vi "Saturation Move Sequence.vi"(2 "error in (no error)":errorcluster, 3 "Saturation Sweep Speed":dbl=2.0, 4 "Saturation End Angle":dbl=320.0, 5 ".NET Refnum in":refnum<k24>) -> (0 "error out":errorcluster, 1 "reference out":refnum<k24>)   [LabVIEW 2023]
uses:
  C:/Users/nanometa/Documents/TCSPC_Git_Repo/Source/ThorLabs.MotionControl.KCube.DCServoCLI.dll
  ThorLabs.MotionControl.KCube.DCServoCLI.dll
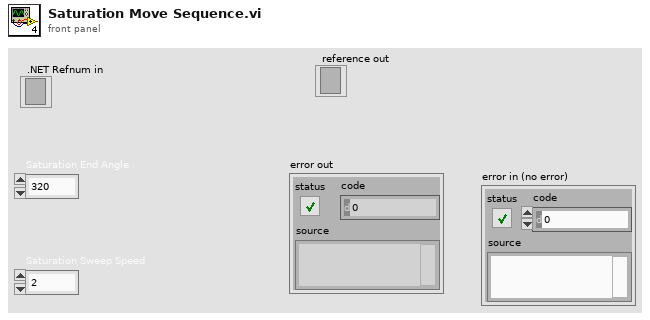
[diagram p1: front panel]
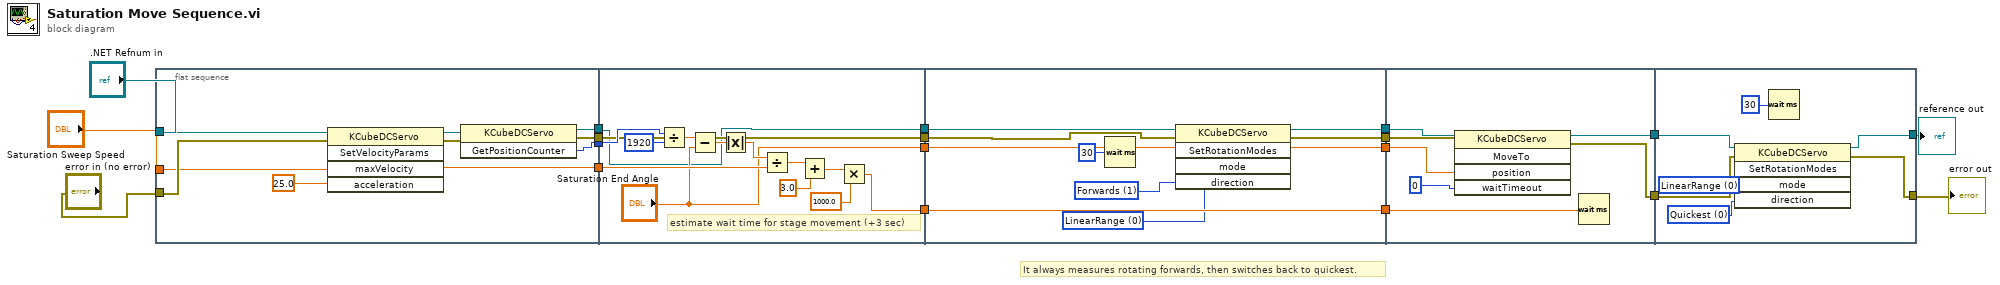
[diagram p0: block diagram]
diagram:
  # "It always measures rotating forwards, then switches back to quickest."
  n1 = flat-sequence {
    tunnel: [w27] -> w19
    tunnel: [w21] -> w18
    tunnel: [w25] -> w17
    tunnel: [w23] -> w16
    tunnel: "error in (no error)" -> [w22]
    tunnel: "Saturation Sweep Speed" -> [w21]
    tunnel: ".NET Refnum in" -> [w20]
    tunnel: w19 -> [w33]
    tunnel: w18 -> [w38]
    tunnel: [w32] -> w10
    tunnel: w17 -> [w32]
    tunnel: [w31] -> w8
    tunnel: ["Saturation End Angle"] -> w6
    tunnel: [w29] -> w4
    tunnel: w16 -> [w29]
    tunnel: w10 -> [w46]
    tunnel: [w47] -> w9
    tunnel: w8 -> [w51]
    tunnel: [w51] -> w7
    tunnel: w6 -> [w50]
    tunnel: [w50] -> w5
    tunnel: w4 -> [w49]
    tunnel: [w48] -> w3
    tunnel: w9 -> [w57]
    tunnel: w7 -> [w56]
    tunnel: w5 -> [w55]
    tunnel: w3 -> [w54]
    tunnel: [w53] -> w2
    tunnel: [w52] -> w1
    tunnel: [w60] -> w14
    tunnel: [w61] -> w15
    tunnel: w2 -> [w65]
    tunnel: w1 -> [w64]
    frame #0 {
      n2 = invoke class="KCubeDCServo" method="SetVelocityParams"(reference=w20, error in=w22, "maxVelocity"=w21, "acceleration"=25.0) -> (reference out=w24:refnum<k24>, error out=w26:errorcluster)  [unwired: 1 in, 3 out]
      n3 = invoke class="KCubeDCServo" method="GetPositionCounter"(reference=w24, error in=w26) -> (reference out=w23:refnum<k24>, error out=w25:errorcluster, "GetPositionCounter"=w27:i32)  [unwired: 1 in]
    }
    frame #1 {
      # "estimate wait time for stage movement (+3 sec)"
      n4 = Divide(x=w33, y=1920) -> (x/y=w41:dbl)
      n5 = Subtract(x=w41, y="Saturation End Angle") -> (x-y=w42:dbl)
      n6 = Absolute Value(x=w42) -> (abs(x)=w39:dbl)
      n7 = Divide(x=w39, y=w38) -> (x/y=w37:dbl)
      n8 = Add(x=w37, y=3.0) -> (x+y=w35:dbl)
      n9 = Multiply(x=w35, y=1000.0) -> (x*y=w31:dbl)
    }
    frame #2 {
      w43 = i16 0 items=["LinearRange", "RotationalUnlimited", "RotationalRange"] ("mode")
      w45 = i16 1 items=["Quickest", "Forwards", "Reverse"] ("direction")
      n10 = Wait (ms)(milliseconds to wait=u32 30) -> ()  [unwired: 1 out]
      n11 = invoke class="KCubeDCServo" method="SetRotationModes"(reference=w49, error in=w46, "mode"=w43, "direction"=w45) -> (reference out=w48:refnum<k24>, error out=w47:errorcluster)  [unwired: 1 in, 3 out]
    }
    frame #3 {
      n12 = invoke class="KCubeDCServo" method="MoveTo"(reference=w54, error in=w57, "position"=w55, "waitTimeout"=0) -> (reference out=w53:refnum<k24>, error out=w52:errorcluster)  [unwired: 1 in, 3 out]
      n13 = Wait (ms)(milliseconds to wait=w56) -> ()  [unwired: 1 out]
    }
    frame #4 {
      w59 = i16 0 items=["LinearRange", "RotationalUnlimited", "RotationalRange"] ("mode")
      w63 = i16 0 items=["Quickest", "Forwards", "Reverse"] ("direction")
      n14 = invoke class="KCubeDCServo" method="SetRotationModes"(reference=w65, error in=w64, "mode"=w59, "direction"=w63) -> (reference out=w61:refnum<k24>, error out=w60:errorcluster)  [unwired: 1 in, 3 out]
      n15 = Wait (ms)(milliseconds to wait=u32 30) -> ()  [unwired: 1 out]
    }
  }
  "reference out" <- w15
  "error out" <- w14
